vi "Delete.vi"(8 "error in":errorcluster, 10 "endPoint":string, 11 "firebase in":refnum<class "firebase.lvclass">) -> (0 "error out":errorcluster, 2 "Item":string)   [LabVIEW 2019, in "firebase.lvclass"]
uses:
  firebase.lvclass
  <vilib>/NI/Advanced HTTP Client/Header--Combo Box.ctl
  <vilib>/JDP Science/JSONtext/Next JSON Value.vi
  <vilib>/JDP Science/JSONtext/String Subset.vi
  <vilib>/JDP Science/JSONtext/Parsing/Advance past next JSON Value (inlined COPY).vi
  <vilib>/JDP Science/JSONtext/Parsing/Advance past whitespace.vi
  <vilib>/JDP Science/JSONtext/Parsing/Advance past String.vi
  <vilib>/JDP Science/JSONtext/Parsing/Advance past Number.vi
  <vilib>/JDP Science/JSONtext/Parsing/Advance past Line Ending.vi
  <vilib>/JDP Science/JSONtext/Parsing/Parse Full Path or Item Name.vi
  <vilib>/JDP Science/JSONtext/Parsing/Advance past Array.vi
  <vilib>/JDP Science/JSONtext/Parsing/Advance past Object.vi
  <vilib>/JDP Science/JSONtext/support/Error Cluster From Code.vi
  <vilib>/JDP Science/JSONtext/Offset/Find Item Locations by Path.vi
  <vilib>/NI/Advanced HTTP Client/Session.lvclass
  <vilib>/JDP Science/JSONtext/JSONtext.lvlib
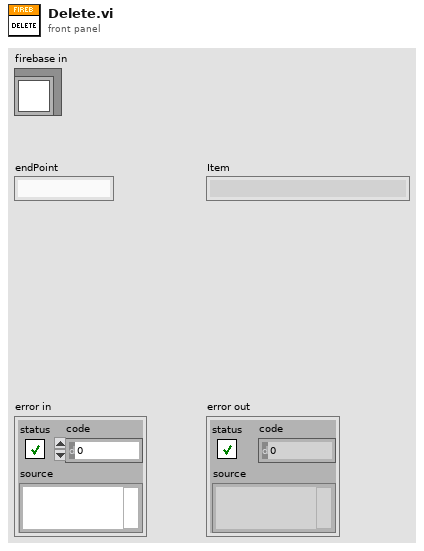
[diagram p1: front panel]
types:
  T1 = typedef "lib_NI_Advanced HTTP Client.lvlib/Session.lvclass/Header--Combo Box.ctl" = string
  T2 = typedef "firebase.lvclass/Success Sign In--cluster.ctl" = cluster{"kind":string, "idToken":string, "email":string, "refreshToken":string, "expiresIn":string, "localId":string, "displayName":string, "registered":bool}
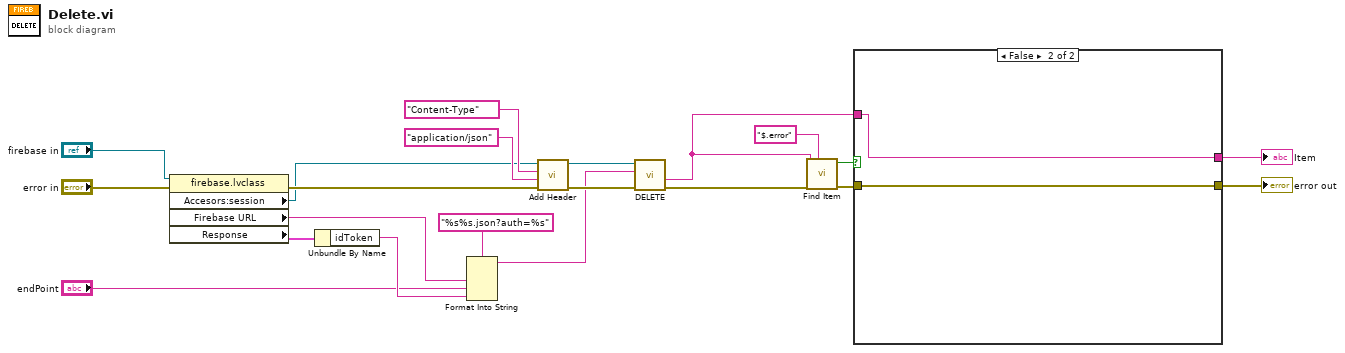
[diagram p0: block diagram]
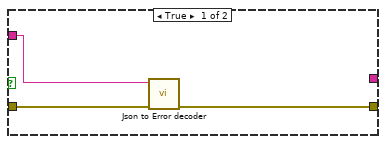
[diagram p2: hidden frame]
diagram:
  n1 = property class="firebase.lvclass"(reference="firebase in", error in="error in") -> (error out=w17:errorcluster, "Accesors:session"=w1:refnum<class "Session.lvclass">, "Firebase URL"=w2:string, "Response"=w6:T2)  [unwired: 1 out]
  n2 = Unbundle By Name(w6) -> ("idToken"=w5:string)
  n3 = Format Into String(format string="%s%s.json?auth=%s", w2, "endPoint", w5) -> (resulting string=w10:string)  [unwired: 2 in, 1 out]
  n4 = call <vilib>:"Add Header.vi"("error in"=w17, "value"="application/json", "header"=T1 "Content-Type", "session in"=w1) -> ("error out"=w19:errorcluster, "session out"=w13:refnum<class "Session.lvclass">)  [unwired: 6 in]
  n5 = call <vilib>:"DELETE.vi"("error in"=w19, "url"=w10, "session in"=w13) -> ("error out"=w20:errorcluster, "body"=w7:string)  [unwired: 4 in, 3 out]
  n6 = call <vilib>:"Find Item.vi"("$Path or Item Name"="$.error", "error in (no error)"=w20, "JSON"=w7) -> ("error out"=w18:errorcluster, "Found"=w8:bool)  [unwired: 5 in, 2 out]
  n7 = case shown="False" w8 {
    tunnel: [w23 w26] -> w16
    tunnel: w18 -> [w24 w26]
    tunnel: w7 -> [w22 w25]
    tunnel: [_ w25] -> w3
    frame True {
      n8 = call "Json to Error decoder.vi"("error in"=w24, "body"=w22) -> ("error out"=w23:errorcluster)  [unwired: 9 in]
    }
    frame False {
    }
  }
  "error out" <- w16
  "Item" <- w3
